vi "Solver.vi"(10 "Word List":string[](array[string]), 11 "Word Search Grid":string[][](array[string])) -> (3 "Solutions":T1)   [LabVIEW 2020]
uses:
  support/Solutions--map.ctl
  support/Letter Index--cluster.ctl
panel:
  # "Implement your Word Search challenge solution in this VI. Do not change the connector pane of this VI."
  # "Letters will always be ALL CAPS."
  # "Words will always be ALL CAPS."
  # "The Word Search Grid contains the 2D array of letters in which all words in the Word List appear. Words can appear forwards, backwards, up, down, and diagonally in any direction.\n\nThe Solutions map will contain one entry per item in the Word List. The map elements are:\n\nWord: The word from the Word List.\nLetter Indices: The row/column indices into the Word Search Grid for each letter (in order) in the word."
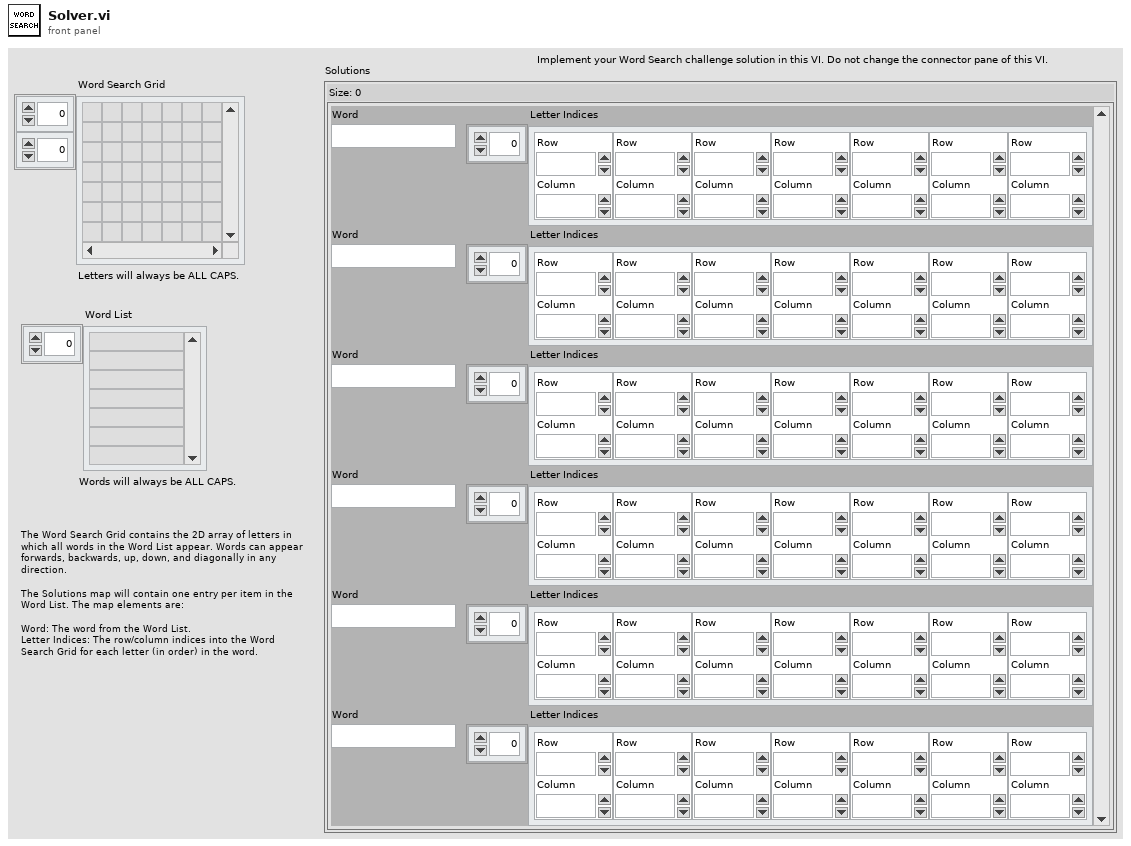
[diagram p1: front panel]
types:
  T1 = typedef "Solutions--map.ctl" = map{string, T2[]}
  T2 = typedef "Letter Index--cluster.ctl" = cluster{"Row":i32, "Column":i32}
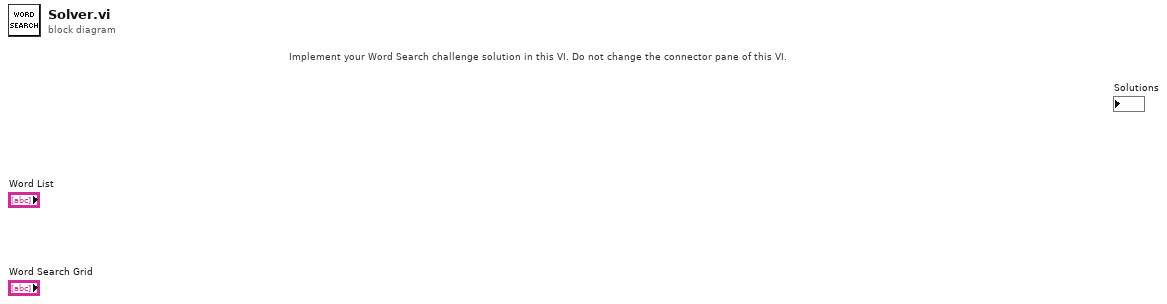
[diagram p0: block diagram]
diagram:
  # "Implement your Word Search challenge solution in this VI. Do not change the connector pane of this VI."
